vi "Hold knobs.vi"(0 "interior circle":refnum<vi>, 1 "middle circle":refnum<vi>, 2 "exterior circle":refnum<vi>) -> ()   [LabVIEW 2010]
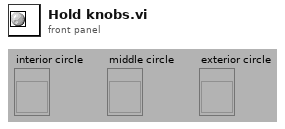
[diagram p1: front panel]
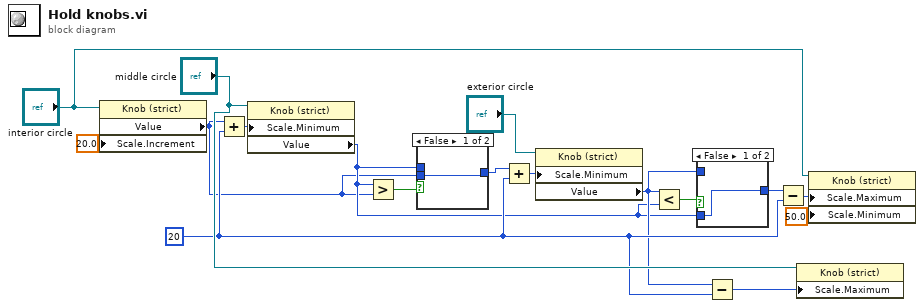
[diagram p0: block diagram]
diagram:
  w14 = i16 20 ("y")
  n1 = property on="Property Node" class="Knob (strict)"(reference="interior circle", "Scale.Increment"=20.0 ("Scale.Range:Increment")) -> ("Value"=w5:i16)  [unwired: 1 in, 2 out]
  n2 = Add(x=w5, y=w14) -> (x+y=w2:i16)
  n3 = property on="Property Node" class="Knob (strict)"(reference="middle circle", "Scale.Minimum"=w2) -> ("Value"=w8:i16)  [unwired: 1 in, 2 out]
  n4 = Greater?(x=w8, y=w5) -> (0:w4:bool)
  n5 = case shown="False" w4 {
    tunnel: w8 -> [_ w19]
    tunnel: [w18 w19] -> w6
    tunnel: w5 -> [w18 _]
    frame False {
    }
    frame True {
    }
  }
  n6 = Add(x=w6, y=w14) -> (x+y=w3:i16)
  n7 = property on="Property Node" class="Knob (strict)"(reference="exterior circle", "Scale.Minimum"=w3) -> ("Value"=w12:i16)  [unwired: 1 in, 2 out]
  n8 = Less?(x=w12, y=w8) -> (x < y?=w7:bool)
  n9 = case shown="False" w7 {
    tunnel: w12 -> [_ w21]
    tunnel: [w20 w21] -> w10
    tunnel: w8 -> [w20 _]
    frame False {
    }
    frame True {
    }
  }
  n10 = Subtract(x=w12, y=w14) -> (x-y=w13:i16)
  n11 = Subtract(x=w10, y=w14) -> (x-y=w9:i16)
  n12 = property on="Property Node" class="Knob (strict)"(reference="middle circle", "Scale.Maximum"=w13) -> ()  [unwired: 1 in, 2 out]
  n13 = property on="Property Node" class="Knob (strict)"(reference="interior circle", "Scale.Maximum"=w9, "Scale.Minimum"=50.0 ("Scale.Range:Minimum")) -> ()  [unwired: 1 in, 2 out]
